vi "Approach_ChargeAccumulator.vi"(7 "Computer called (T/F)":bool) -> ()   [LabVIEW 2023]
uses:
  Settings.vi
  Sub_Vi/TypeDefs/WayPointCluster.ctl
  Sub_Vi/TypeDefs/ChangeOnFly.ctl
  Sub_Vi/TypeDefs/Display.ctl
  Sub_Vi/TypeDefs/Settings.ctl
  Sub_Vi/TypeDefsControls/Zposition.ctl
  Sub_Vi/TypeDefsControls/Piezo Velocity.ctl
  Sub_Vi/TypeDefsControls/Voltage.ctl
  Sub_Vi/TypeDefsControls/Feedback Type.ctl
  Sub_Vi/TypeDefsControls/Xposition.ctl
  Sub_Vi/TypeDefsControls/Yposition.ctl
panel:
  in  "Charge Accumulator (q)":dbl
  in  "Tab Control 2":T1(tab)
  out "C1":dbl[](graph)
  out "C2":dbl[](graph)
  out "C3":dbl[](graph)
  in  "Feedback Type":T2=enum."Current 1"
  in  "Tab Control":enum32{"C1 vs Z", "C2 vs Z", "C3 vs Z"}(tab)
  out "Z vs C1":cluster{"Y":dbl[], "Y":dbl[]}[](graph)
  out "Z vs C2":cluster{"Y":dbl[], "Y":dbl[]}[](graph)
  out "Z vs C3":cluster{"Y":dbl[], "Y":dbl[]}[](graph)
  in  "SettingsCluster":T3={"Sample Rate (us)"=1, "Samples Per Data Point (int, power of 2)"=1000, "DistanceToBulk (um)"=-1.0, "HoldTimeScaler"=1, "SaveData"=TRUE, "DistanceToBulk (um) 2"=-1.0, "DistanceToBulk (um) 3"=-1.0}
  in  "Display Cluster":T4
  in  "ChangeonFly":T5
  in  "WayPointCluster":T6
  in  "Start scan Button":bool
  in  "Stop":bool
  in  "Pause":bool
  in  "Greater Than":bool=TRUE
  in  "Set X":bool
  in  "Set Y":bool
  in  "Y":T7=50.0 min=0.0 max=100000.0
  in  "X":T8=50.0 min=0.0 max=100000.0
  in  "Retract after approach":bool=TRUE
  in  "Approach Voltage (V)":T9=0.35 min=-10.0 max=10.0
  in  "Approach Rate (µm/s)":T10=0.1 min=0.0
  in  "End Extension (µm)":T11 min=0.0 max=100000.0
  in  "Start Extention (µm)":T11=150.0 min=0.0 max=100000.0
  in  "Feedback Threshold (A)":dbl
  in  "Start Scanning Button":bool
  out "Lockin Phase":dbl[](graph)
  out "Lockin Amp":dbl[](graph)
  # "Settings"
  # "Pause at"
  # "Advanced Settings"
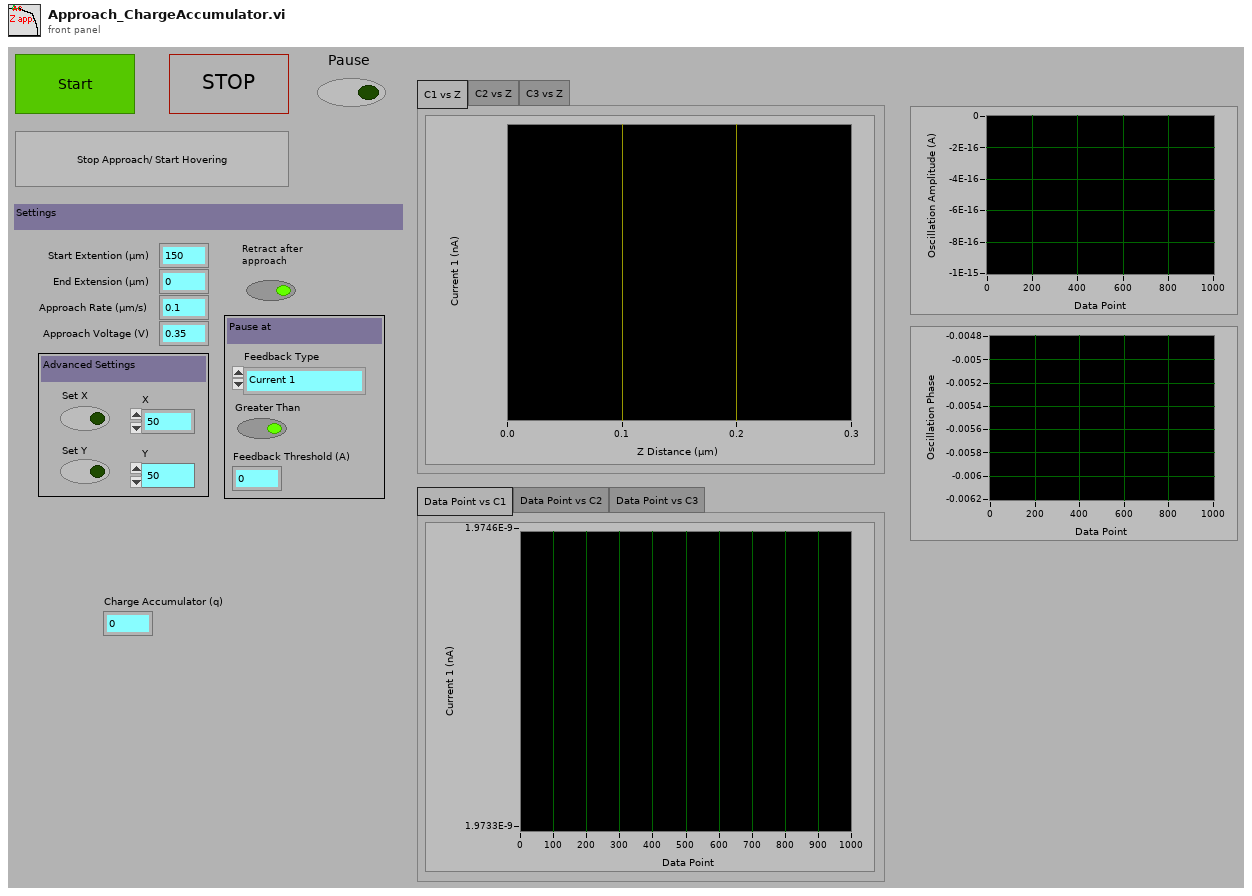
[diagram p1: front panel]
types:
  T1 = enum32{"Data Point vs C1", "Data Point vs C2", "Data Point vs C3"}
  T2 = typedef "Feedback Type.ctl" = enum16{"AC Magnitude", "Current 1", "Current 2", "Phase"}
  T3 = typedef "Settings.ctl" = cluster{"Sample Rate (us)":u32, "Samples Per Data Point (int, power of 2)":i16, "DistanceToBulk (um)":dbl, "HoldTimeScaler":u64, "SaveData":bool, "DistanceToBulk (um) 2":dbl, "DistanceToBulk (um) 3":dbl}
  T4 = typedef "Display.ctl" = cluster{"X":refnum<vi>, "Y":refnum<vi>, "Z":refnum<vi>, "Amp":refnum<vi>, "Phase":refnum<vi>, "t vs Z":refnum<vi>, "t vs C1":refnum<vi>, "t vs C2":refnum<vi>, "t vs C3":refnum<vi>, "t vs Amp":refnum<vi>, "t vs Phase":refnum<vi>, "t vs X":refnum<vi>, "t vs Y":refnum<vi>, "Z vs C1":refnum<vi>, "Z vs C2":refnum<vi>, "Z vs C3":refnum<vi>, "V vs C1":refnum<vi>, "V vs C2":refnum<vi>, "V vs C3":refnum<vi>, "X/Y/Z F":refnum<vi>, "X/Y/Z R":refnum<vi>, "X/Y/C1 F":refnum<vi>, "X/Y/C1 R":refnum<vi>, "X/Y/C2 F":refnum<vi>, "X/Y/C2 R":refnum<vi>, "X/Y/C3 F":refnum<vi>, "X/Y/C3 R":refnum<vi>, "NumberOfLines":u16, "um Per Pixel":dbl, "um Per Line":dbl, "X Center":dbl, "Hop X/Y/Z":refnum<vi>, "Hop X/Y/C1":refnum<vi>, "Hop X/Y/C2":refnum<vi>, "Hop X/Y/C3":refnum<vi>, "X Width":dbl, "Y Width":dbl, "Hopping Distance":dbl, "V2 vs C1":refnum<vi>, "V vs Phase":refnum<vi>, "Y Center":dbl, "Number of Pixels":dbl, "V2 vs C2":refnum<vi>, "V2 vs C3":refnum<vi>, "V vs y":refnum<vi>, "V2 vs y":refnum<vi>, "Z vs Amp":refnum<vi>, "Z vs Phase":refnum<vi>}
  T5 = typedef "ChangeOnFly.ctl" = cluster{"Stop (boolean)":refnum<vi>, "Pause (boolean)":refnum<vi>, "EndCurrentLine (boolean)":refnum<vi>, "max movement per update step (Interger, nm)":refnum<vi>, "P (float, arb)":refnum<vi>, "Feedback set point (double, Amps)":refnum<vi>, "Voltage (double, V)":refnum<vi>, "Feedback set point 2 (double, Amps)":refnum<vi>, "Stop on Greater Than 2? (boolean)":refnum<vi>, "Stop on Greater Than? (boolean)":refnum<vi>, "Voltage 2 (double, V)":refnum<vi>, "Feedback Type (enum)":refnum<vi>, "Feedback Type 2 (enum)":refnum<vi>}
  T6 = typedef "WayPointCluster.ctl" = cluster{"X (um)":dbl[], "Y (um)":dbl[], "Z (um)":dbl[], "V (V)":dbl[], "X Velocity (um s-1)":dbl[], "Y Velocity (um s-1)":dbl[], "Z Velocity (um s-1)":dbl[], "V Velocity (V s-1)":dbl[], "FeedBack Type (enum)":u16[], "Move X (boolean)":bool[], "Move Y (boolean)":bool[], "Move Z (boolean)":bool[], "Move V (boolean)":bool[], "Jump V (boolean)":bool[], "Hold (boolean)":bool[], "Hold Time":u32[], "V2 (V)":dbl[], "Move V2":bool[], "V2 Velocity (V s-1)":dbl[], "Jump V2 (boolean)":bool[], "Update z Position delta (ms)":i16[], "Hold Feedback1":bool[], "Move Z PicoMotor":bool[], " Z PicoMotor Direction":bool[], "DIO0":bool[]}
  T7 = typedef "Yposition.ctl" = dbl
  T8 = typedef "Xposition.ctl" = dbl
  T9 = typedef "Voltage.ctl" = dbl
  T10 = typedef "Piezo Velocity.ctl" = dbl
  T11 = typedef "Zposition.ctl" = dbl
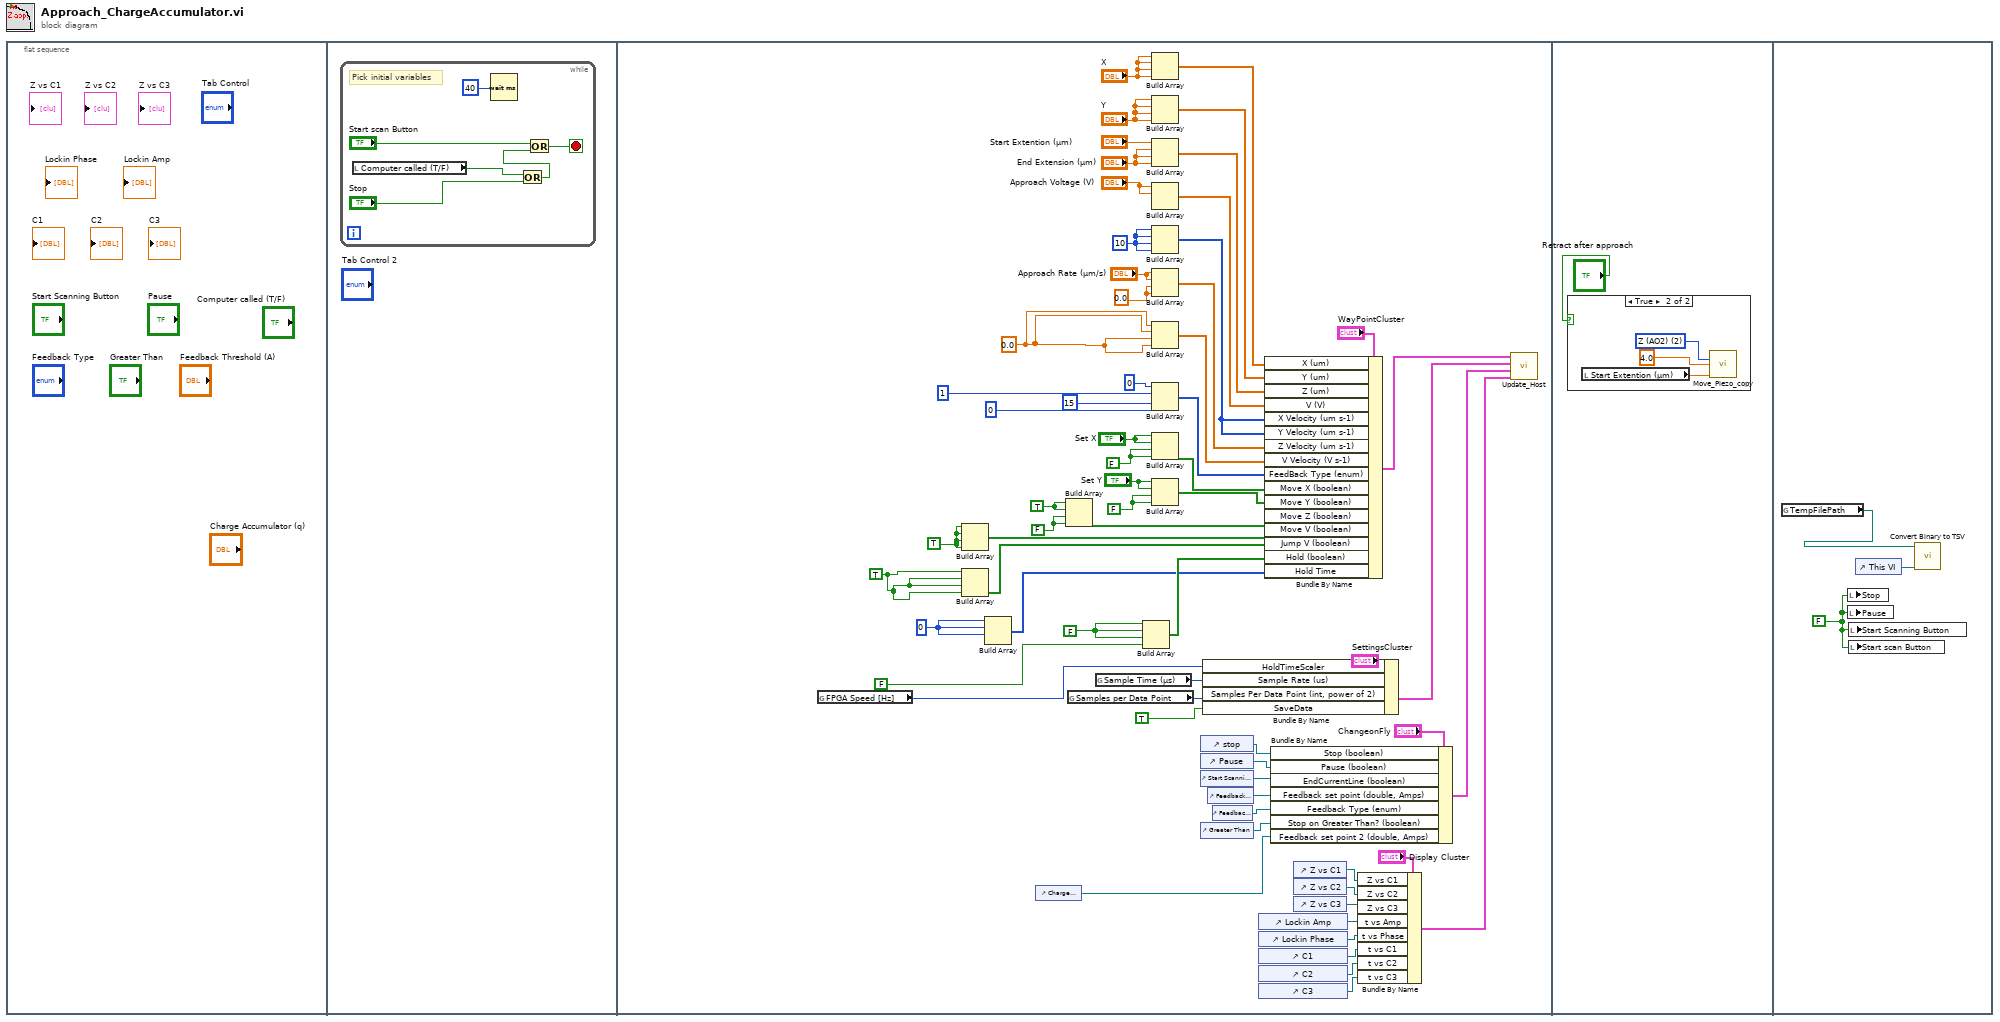
[diagram p0: block diagram]
diagram:
  n1 = flat-sequence {
    frame #0 {
    }
    frame #1 {
      n2 = while {
        stop <- w6 stop-if-true
        # "Pick initial variables"
        n3 = local read "Computer called (T/F)"() -> (w1:bool)
        n4 = Wait (ms)(milliseconds to wait=u32 40) -> ()  [unwired: 1 out]
        n5 = Or(x=w1, y="Stop") -> (x .or. y?=w2:bool)
        n6 = Or(x="Start scan Button", y=w2) -> (x .or. y?=w6:bool)
      }
    }
    frame #2 {
      w49 = u32 0 ("element")
      w13 = TRUE ("Set Z")
      w18 = TRUE ("element")
      w50 = FALSE ("element")
      w53 = FALSE ("element")
      w54 = FALSE ("element")
      w12 = 0.0
      w24 = 0.0 ("element")
      w15 = FALSE ("Set Z")
      w59 = TRUE ("Set Z")
      w52 = 10
      n7 = global read "Settings.vi" "FPGA Speed [Hz]"() -> (w11:i64)
      n8 = Build Array(w18, w18, w18, w18) -> (w19:bool[])
      n9 = Build Array(w13, w13, w13, w13) -> (w64:bool[])
      n10 = Build Array(w49, w49, w49) -> (w62:u32[])  [unwired: 1 in]
      n11 = control-ref of="Charge Accumulator (q)"() -> (w7:refnum<vi>)
      n12 = Build Array(w59, w59, w50, w50) -> (w51:bool[])
      n13 = global read "Settings.vi" "Samples per Data Point"() -> (w57:u16)
      n14 = global read "Settings.vi" "Sample Time (µs)"() -> (w58:u32)
      n15 = Build Array(w15, w15, w15, FALSE ("Set Z")) -> (w67:bool[])
      n16 = Build Array("X", "X", "X", "X") -> (w72:T8[])
      n17 = Build Array("Y", "Y", "Y", "Y") -> (w71:T7[])
      n18 = Build Array("Start Extention (µm)", "End Extension (µm)", "End Extension (µm)", "End Extension (µm)") -> (w16:T11[])
      n19 = Build Array("Approach Voltage (V)", "Approach Voltage (V)", w26) -> (w55:T9[], w26:T9)
      n20 = Build Array(w52, w52, w52, w52) -> (w73:i32[])
      n21 = Build Array("Approach Rate (µm/s)", "Approach Rate (µm/s)", w24, w24) -> (w70:T10[])
      n22 = Build Array(w12, w12, w12, w12) -> (w66:dbl[])
      n23 = Build Array(u16 0 ("element"), u16 1, u16 15 ("element"), u16 0 ("element")) -> (w65:u16[])
      n24 = Build Array("Set X", "Set X", w53, w53) -> (w69:bool[])
      n25 = Build Array("Set Y", "Set Y", w54, w54) -> (w17:bool[])
      n26 = control-ref of="stop"() -> (w33:refnum<vi>)
      n27 = control-ref of="Pause"() -> (w34:refnum<vi>)
      n28 = control-ref of="Start Scanning Button"() -> (w35:refnum<vi>)
      n29 = control-ref of="Greater Than"() -> (w37:refnum<vi>)
      n30 = Bundle By Name(cluster="SettingsCluster", "HoldTimeScaler"=w11, "Sample Rate (us)"=w58, "Samples Per Data Point (int, power of 2)"=w57, "SaveData"=TRUE) -> (w68:T3)
      n31 = control-ref of="Feedback Threshold (A)"() -> (w38:refnum<vi>)
      n32 = control-ref of="Feedback Type"() -> (w36:refnum<vi>)
      n33 = control-ref of="Lockin Amp"() -> (w47:refnum<vi>)
      n34 = control-ref of="Lockin Phase"() -> (w46:refnum<vi>)
      n35 = control-ref of="C1"() -> (w43:refnum<vi>)
      n36 = control-ref of="C2"() -> (w42:refnum<vi>)
      n37 = control-ref of="C3"() -> (w41:refnum<vi>)
      n38 = Bundle By Name(cluster="WayPointCluster", "X (um)"=w72, "Y (um)"=w71, "Z (um)"=w16, "V (V)"=w55, "X Velocity (um s-1)"=w73, "Y Velocity (um s-1)"=w73, "Z Velocity (um s-1)"=w70, "V Velocity (V s-1)"=w66, "FeedBack Type (enum)"=w65, "Move X (boolean)"=w69, "Move Y (boolean)"=w17, "Move Z (boolean)"=w51, "Move V (boolean)"=w19, "Jump V (boolean)"=w64, "Hold (boolean)"=w67, "Hold Time"=w62) -> (w31:T6)
      n39 = Bundle By Name(cluster="ChangeonFly", "Stop (boolean)"=w33, "Pause (boolean)"=w34, "EndCurrentLine (boolean)"=w35, "Feedback set point (double, Amps)"=w38, "Feedback Type (enum)"=w36, "Stop on Greater Than? (boolean)"=w37, "Feedback set point 2 (double, Amps)"=w7) -> (w39:T5)
      n40 = control-ref of="Z vs C1"() -> (w61:refnum<vi>)
      n41 = control-ref of="Z vs C2"() -> (w45:refnum<vi>)
      n42 = control-ref of="Z vs C3"() -> (w44:refnum<vi>)
      n43 = Bundle By Name(cluster="Display Cluster", "Z vs C1"=w61, "Z vs C2"=w45, "Z vs C3"=w44, "t vs Amp"=w47, "t vs Phase"=w46, "t vs C1"=w43, "t vs C2"=w42, "t vs C3"=w41) -> (w30:T4)
      n44 = call "Update_Host.vi"("Display Cluster"=w30, "ChangeonFly"=w39, "SettingsCluster"=w68, "WayPointCluster"=w31) -> ()  [unwired: 6 in]
    }
    frame #3 {
      n45 = case shown="True" "Retract after approach" {
        frame False {
        }
        frame True {
          w77 = u16 2 items=["X (AO0)", "Y (AO1)", "Z (AO2)", "V (AO3)"] ("Channel")
          n46 = local read "Start Extention (µm)"() -> (w75:T11)
          n47 = call "Move_Piezo_copy.vi"("Piezo"=w77, "Movement Speed (µm/s)"=4.0 ("Scan Rate (um/s)"), "Position (µm) (or V)"=w75) -> ()  [unwired: 13 in]
        }
      }
    }
    frame #4 {
      w79 = FALSE ("stop recording")
      n48 = global read "Settings.vi" "TempFilePath"() -> (w78:path)
      n49 = local write "Stop"(w79) -> ()
      n50 = local write "Pause"(w79) -> ()
      n51 = local write "Start Scanning Button"(w79) -> ()
      n52 = local write "Start scan Button"(w79) -> ()
      n53 = control-ref of="This VI"() -> (w80:refnum<vi>)
      n54 = call "Convert Binary to TSV.vi"("This VI"=w80, "TDMS DataFile Name"=w78) -> ()  [unwired: 10 in]
    }
  }
